vi "Get Current Positions.vi"(8 "error in (no error)":errorcluster, 10 "Array of axes":T1[](array[typedef]), 11 "VISA in":refnum<visa-resource-name>) -> (0 "error out":errorcluster, 2 "Array of positions [internal units]":dbl[](array[numeric]), 3 "VISA out":refnum<visa-resource-name>)   [LabVIEW 2018, in "ASI TG-1000.lvlib"]
doc: "Queries the ASI controller for the current position of the specified axes; the equivalent of the WHERE command."
uses:
  ASI TG-1000.lvlib
  Utility/Axis Name.ctl
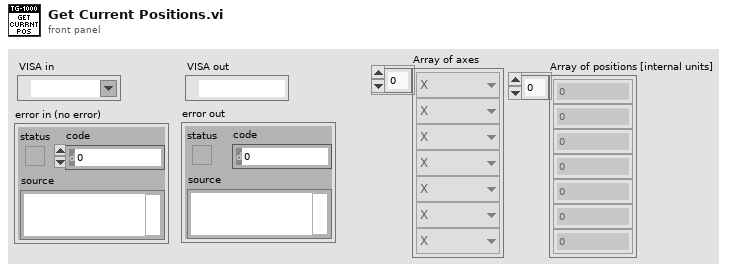
[diagram p1: front panel]
types:
  T1 = typedef "ASI TG-1000.lvlib/Axis Name.ctl" = enum8{"undefined", "A", "B", "C", "D", "E", "F", "G", "H", "I", "J", "K", "L", "M", "N", "O", "P", "Q", "R", "S", "T", "U", "V", "W", "X", "Y", "Z"}
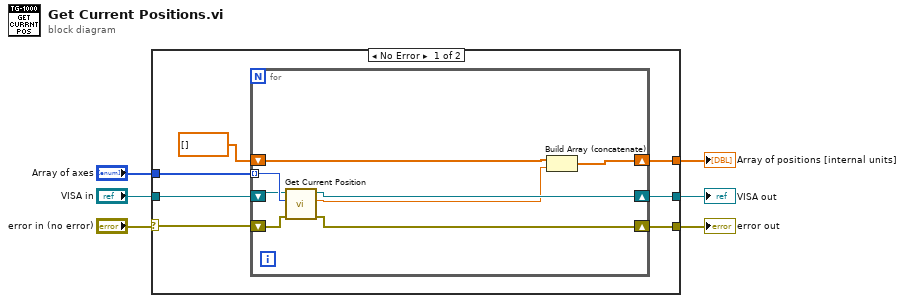
[diagram p0: block diagram]
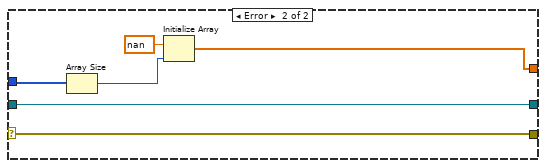
[diagram p2: hidden frame]
diagram:
  n1 = case shown="No Error" "error in (no error)" {
    selector: "error in (no error)" -> [w9 w27]
    tunnel: "VISA in" -> [w13 w26]
    tunnel: [w12 w26] -> w5
    tunnel: [w11 w27] -> w4
    tunnel: "Array of axes" -> [w10 w25]
    tunnel: [w7 w22] -> w1
    frame No Error {
      n2 = for {
        shift-right: [w17] -> w12
        shift-left: w13 -> [w18]
        shift-right: [w20] -> w11
        shift-left: w9 -> [w21]
        tunnel: w10 -> [w19] mode=indexing
        shift-right: [w14] -> w7
        shift-left: dbl[] [] -> [w15]
        n3 = call "Get Current Position.vi"("error in (no error)"=w21, "Axis"=w19, "VISA in"=w18) -> ("error out"=w20:errorcluster, "position [internal units]"=w16:dbl, "VISA out"=w17:refnum<visa-resource-name>)  [unwired: 6 in]
        n4 = Build Array (concatenate)(w15, w16) -> (w14:dbl[])
      }
    }
    frame Error {
      n5 = Array Size(array=w25) -> (size(s)=w23:i32)
      n6 = Initialize Array(nan ("element"), w23) -> (w22:dbl[])
    }
  }
  "VISA out" <- w5
  "error out" <- w4
  "Array of positions [internal units]" <- w1
